vi "SMTP Email Get Token Line.vi"(2 "Offset":i32, 3 "string":string) -> (0 "line len":i32, 1 "Line":string)   [LabVIEW 2012, in "NewNI_SMTPEmail.lvlib"]
uses:
  NewNI_SMTPEmail.lvlib
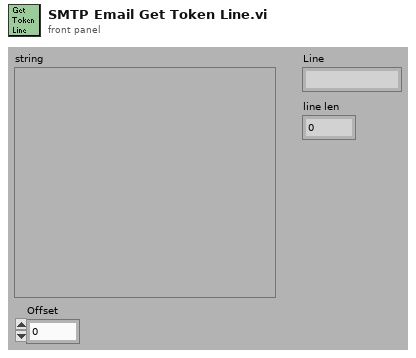
[diagram p1: front panel]
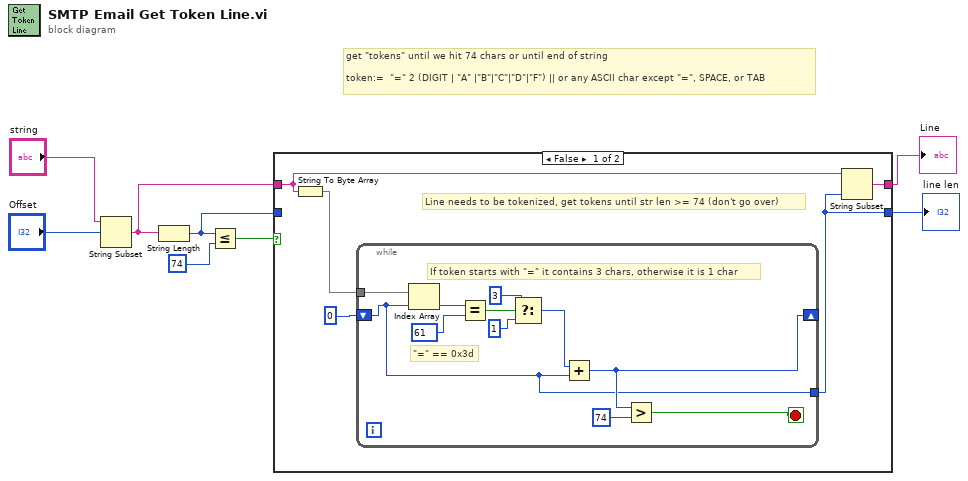
[diagram p0: block diagram]
diagram:
  # "get \"tokens\" until we hit 74 chars or until end of string\n\ntoken:=  \"=\" 2 (DIGIT | \"A\" |\"B\"|\"C\"|\"D\"|\"F\") || or any ASCII char except \"=\", SPACE, or TAB"
  n1 = String Subset(string="string", offset (0)="Offset") -> (substring=w1:string)  [unwired: 1 out]
  n2 = String Length(string=w1) -> (length=w3:i32)
  n3 = Less Or Equal?(x=w3, y=74) -> (x <= y?=w7:bool)
  n4 = case shown="False" w7 {
    tunnel: w1 -> [w10 w26]
    tunnel: [w9 w26] -> w5
    tunnel: w3 -> [_ w25]
    tunnel: [w11 w25] -> w2
    frame False {
      # "Line needs to be tokenized, get tokens until str len >= 74 (don't go over)"
      n5 = String To Byte Array(string=w10) -> (unsigned byte array=w13:u8[])
      n6 = while {
        tunnel: w13 -> [w24]
        shift-right: [w17] -> _
        shift-left: 0 -> [w14]
        tunnel: [w14] -> w11
        stop <- w15 stop-if-true
        # "If token starts with \"=\" it contains 3 chars, otherwise it is 1 char"
        # "\"=\" == 0x3d"
        n7 = Index Array(array=w24, index=w14) -> (element=w23:u8)
        n8 = Equal?(x=w23, y=u8 61) -> (x = y?=w21:bool)
        n9 = Select(t=3, s=w21, f=1) -> (s? t:f=w18:i32)
        n10 = Add(x=w18, y=w14) -> (x+y=w17:i32)
        n11 = Greater?(x=w17, y=74) -> (0:w15:bool)
      }
      n12 = String Subset(string=w10, length (rest)=w11) -> (substring=w9:string)  [unwired: 1 out]
    }
    frame True {
      # "Substring is short enough return the whole string"
    }
  }
  "Line" <- w5
  "line len" <- w2
